vi "Db PXI8431 process.vi"(8 "error in (no error)":errorcluster, 10 "UIname":string="PXI8431_7_com_slot7.vi", 11 "VI in":refnum<vi>) -> (0 "error out":errorcluster, 2 "Boolean":bool, 3 "VI out":refnum<vi>)   [LabVIEW 2017]
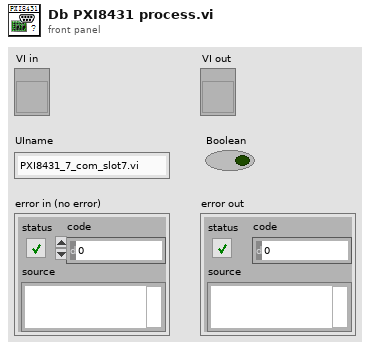
[diagram p1: front panel]
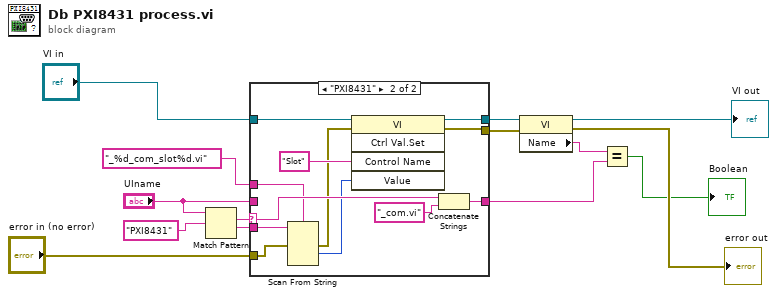
[diagram p0: block diagram]
diagram:
  n1 = Match Pattern(string="UIname", regular expression="PXI8431") -> (match substring=w10:string, after substring=w3:string)  [unwired: 1 in, 2 out]
  n2 = case shown="\"PXI8431\"" w10 {
    selector: w10 -> [_ w28]
    tunnel: "UIname" -> [w17 _]
    tunnel: [w17 w29] -> w5
    tunnel: "VI in" -> [w16 w26]
    tunnel: [w16 w25] -> w6
    tunnel: "error in (no error)" -> [w15 w19]
    tunnel: [w15 w24] -> w4
    tunnel: w3 -> [_ w22]
    tunnel: "_%d_com_slot%d.vi" -> [_ w21]
    frame "", Default {
    }
    frame "PXI8431" {
      n3 = Scan From String(format string=w21, input string=w22, error in=w19) -> (error out=w18:errorcluster, output 1=w20:i32)  [unwired: 4 in, 2 out]
      n4 = invoke class="VI" method="Ctrl Val.Set"(reference=w26, error in=w18, "Control Name"="Slot", "Value"=w20) -> (reference out=w25:refnum<vi>, error out=w24:errorcluster)  [unwired: 1 in, 3 out]
      n5 = Concatenate Strings(w28, "_com.vi") -> (w29:string)
    }
  }
  n6 = property class="VI"(reference=w6, error in=w4) -> (reference out=→"VI out":refnum<vi>, error out=→"error out":errorcluster, "Name"=w12:string)
  n7 = Equal?(x=w12, y=w5) -> (x = y?=→"Boolean":bool)
